vi "Get Config Path.vi"(11 "Output Actor Hardware Interface.lvclass":refnum<class "Output Actor Hardware Interface.lvclass">) -> (2 "Path":path, 3 "Output Actor Hardware Interface.lvclass 2":refnum<class "Output Actor Hardware Interface.lvclass">)   [LabVIEW 2015, in "Output Actor Hardware Interface.lvclass"]
uses:
  Output Actor Hardware Interface.lvclass
  Output Actor Hardware Interface.lvclass/Output Actor Hardware Interface.ctl
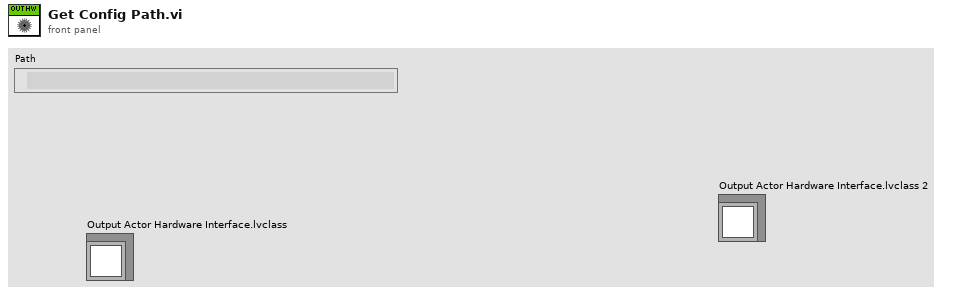
[diagram p1: front panel]
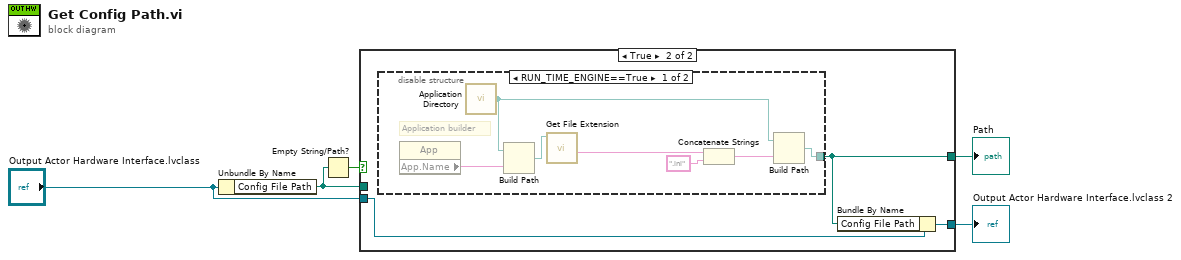
[diagram p0: block diagram]
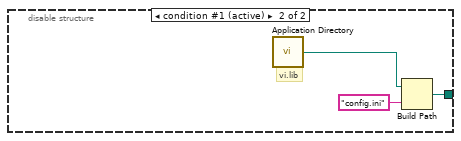
[diagram p3: hidden frame]
diagram:
  n1 = Unbundle By Name("Output Actor Hardware Interface.lvclass") -> ("Config File Path"=w2:path)
  n2 = Empty String/Path?(string/path=w2) -> (empty?=w5:bool)
  n3 = case shown="True" w5 {
    tunnel: [w7 w9] -> w1
    tunnel: w2 -> [w7 _]
    tunnel: [w6 w8] -> w4
    tunnel: "Output Actor Hardware Interface.lvclass" -> [w6 w10]
    frame False {
    }
    frame True {
      n4 = disable-structure shown="RUN_TIME_ENGINE==True" {
        disable-tunnel: [w12 w18] -> w9
        frame condition #0 {
          # "Application builder"
          n5 = property class="App"() -> ("App.Name"=w17:string)  [unwired: 2 in, 2 out]
          n6 = call <vilib>:"Application Directory.vi"() -> ("Application Directory"=w11:path)
          n7 = Build Path(base path=w11, name or relative path=w17) -> (appended path=w13:path)
          n8 = call <vilib>:"Get File Extension.vi"("file"=w13) -> ("filename without extension"=w16:string)  [unwired: 6 in, 4 out]
          n9 = Concatenate Strings(w16, ".ini" ("string")) -> (w14:string)
          n10 = Build Path(base path=w11, name or relative path=w14) -> (appended path=w12:path)
        }
        frame condition #1 (active) {
          # "vi.lib"
          n11 = call <vilib>:"Application Directory.vi"() -> ("Application Directory"=w19:path)
          n12 = Build Path(base path=w19, name or relative path="config.ini") -> (appended path=w18:path)
        }
      }
      n13 = Bundle By Name(cluster=w10, "Config File Path"=w9) -> (w8:refnum<class "Output Actor Hardware Interface.lvclass">)
    }
  }
  "Path" <- w1
  "Output Actor Hardware Interface.lvclass 2" <- w4
